vi "Get Ls1 control refums.vi"(11 "UI ctrl refs":T1) -> (1 "Ls1Shutter":refnum<vi>, 2 "Ls1 Confirm Wav":refnum<vi>, 3 "Digital out":refnum<vi>)   [LabVIEW 2017]
uses:
  Typedefs/UI ctrl refs cluster.ctl
  Typedefs/Laser control knob.ctl
  Typedefs/Frame Size.ctl
  Typedefs/Plane Mode.ctl
  Typedefs/PMT control knob.ctl
  Typedefs/XY Stage_Move.ctl
  User Interface/Misc/Experiment Type.ctl
  User Interface/Misc/Biology Information.ctl
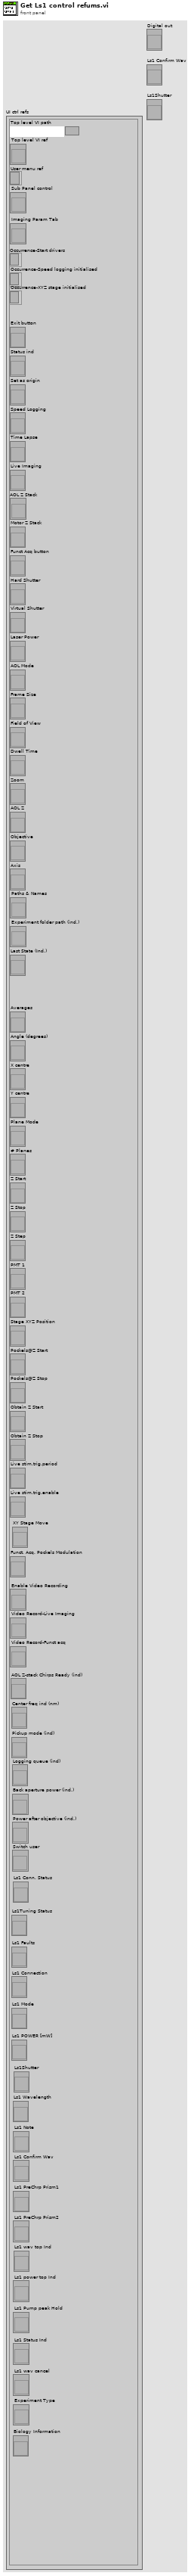
[diagram p1: front panel]
types:
  T1 = typedef "UI ctrl refs cluster.ctl" = cluster{"Top level VI path":path, "Top level VI ref":refnum<vi>, "User menu ref":refnum<k9>, "Sub Panel control":refnum<vi>, "Imaging Param Tab":refnum<vi>, "Occurrence-Start drivers":refnum<k4>, "Occurrence-Speed logging initialised":refnum<k4>, "Occurrence-XYZ stage initialised":refnum<k4>, "Exit button":refnum<vi>, "Status ind":refnum<vi>, "Set as origin":refnum<vi>, "Speed Logging":refnum<vi>, "Time Lapse":refnum<vi>, "Live Imaging":refnum<vi>, "AOL Z Stack":refnum<vi>, "Motor Z Stack":refnum<vi>, "Funct Acq button":refnum<vi>, "Hard Shutter":refnum<vi>, "Virtual Shutter":refnum<vi>, "Laser Power":refnum<vi>, "AOL Mode":refnum<vi>, "Frame Size":refnum<vi>, "Field of View":refnum<vi>, "Dwell Time":refnum<vi>, "Zoom":refnum<vi>, "AOL Z":refnum<vi>, "Objective":refnum<vi>, "Axis":refnum<vi>, "Paths & Names":refnum<vi>, "Experiment folder path (ind.)":refnum<vi>, "Last State (Ind.)":refnum<vi>, "Averages":refnum<vi>, "Angle (degrees)":refnum<vi>, "X centre":refnum<vi>, "Y centre":refnum<vi>, "Plane Mode":refnum<vi>, "# Planes":refnum<vi>, "Z Start":refnum<vi>, "Z Stop":refnum<vi>, "Z Step":refnum<vi>, "PMT 1":refnum<vi>, "PMT 2":refnum<vi>, "Stage XYZ Position":refnum<vi>, "Pockels@Z Start":refnum<vi>, "Pockels@Z Stop":refnum<vi>, "Obtain Z Start":refnum<vi>, "Obtain Z Stop":refnum<vi>, "Live stim.trig.period":refnum<vi>, "Live stim.trig.enable":refnum<vi>, "XY Stage Move":refnum<vi>, "Funct. Acq. Pockels Modulation":refnum<vi>, "Enable Video Recording":refnum<vi>, "Video Record-Live Imaging":refnum<vi>, "Video Record-Funct acq":refnum<vi>, "AOL Z-stack Chirps Ready (ind)":refnum<vi>, "Center freq ind (nm)":refnum<vi>, "Pickup mode (ind)":refnum<vi>, "Logging queue (ind)":refnum<vi>, "Back aperture power (ind.)":refnum<vi>, "Power after objective (ind.)":refnum<vi>, "Switch user":refnum<vi>, "Ls1 Conn. Status":refnum<vi>, "Ls1Tuning Status":refnum<vi>, "Ls1 Faults":refnum<vi>, "Ls1 Connection":refnum<vi>, "Ls1 Mode":refnum<vi>, "Ls1 POWER [mW]":refnum<vi>, "Ls1Shutter":refnum<vi>, "Ls1 Wavelength":refnum<vi>, "Ls1 Note":refnum<vi>, "Ls1 Confirm Wav":refnum<vi>, "Ls1 PreChrp Prism1":refnum<vi>, "Ls1 PreChrp Prism2":refnum<vi>, "Ls1 wav top Ind":refnum<vi>, "Ls1 power top Ind":refnum<vi>, "Ls1 Pump peak Hold":refnum<vi>, "Ls1 Status Ind":refnum<vi>, "Ls1 wav cancel":refnum<vi>, "Experiment Type":refnum<vi>, "Biology Information":refnum<vi>}
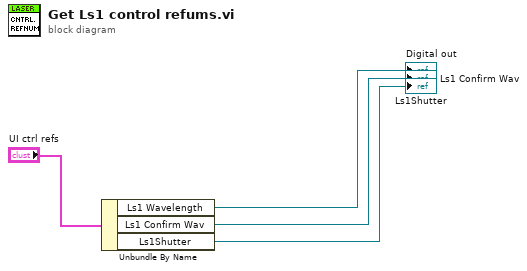
[diagram p0: block diagram]
diagram:
  n1 = Unbundle By Name("UI ctrl refs") -> ("Ls1 Wavelength"=→"Digital out":refnum<vi>, "Ls1 Confirm Wav"=→"Ls1 Confirm Wav":refnum<vi>, "Ls1Shutter"=→"Ls1Shutter":refnum<vi>)
